vi "Check Value Type.vi"(8 "error in (no error)":errorcluster, 11 "Column in":refnum<class "Column Parent.lvclass">) -> (0 "error out":errorcluster, 3 "Column out":refnum<class "Column Parent.lvclass">)   [LabVIEW 2020, in "Basic Columns.lvlib" / "Column Parent.lvclass"]
uses:
  Column Parent.lvclass
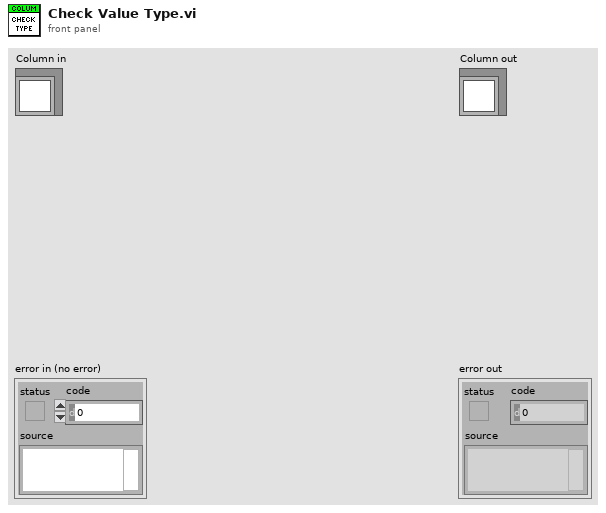
[diagram p1: front panel]
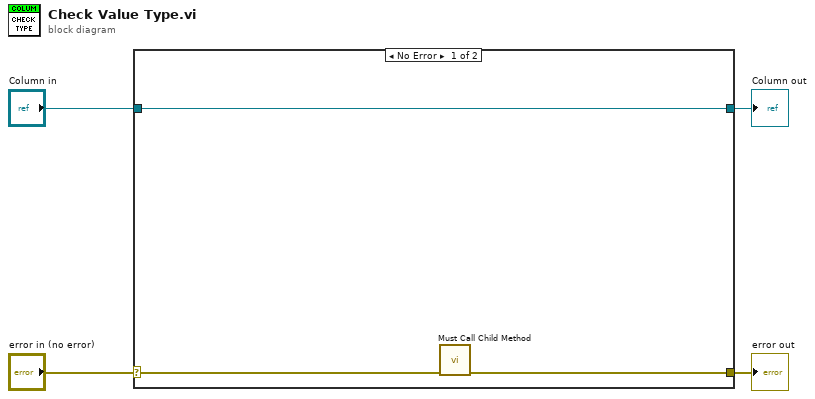
[diagram p0: block diagram]
diagram:
  n1 = case shown="No Error" "error in (no error)" {
    selector: "error in (no error)" -> [w6 w9]
    tunnel: [w5 w9] -> w3
    tunnel: [w7 w8] -> w1
    tunnel: "Column in" -> [w7 w8]
    frame No Error {
      n2 = call "Must Call Child Method.vi"("error in"=w6) -> ("error out"=w5:errorcluster)  [unwired: 10 in]
    }
    frame Error {
    }
  }
  "error out" <- w3
  "Column out" <- w1
